vi "Set Connection Status.vi"(8 "error in (no error)":errorcluster, 10 "Connection Status":T1, 11 "S7NetCom in":refnum<class "S7NetCom.lvclass">) -> (0 "error out":errorcluster, 3 "S7NetCom out":refnum<class "S7NetCom.lvclass">)   [LabVIEW 2014, in "S7NetCom.lvclass"]
doc: "____\nCopyright (c) 2019 Hampel Software Engineering (HSE), released under BSD license. More info can be found on https://dokuwiki.hampel-soft.com/code/hse/s7netcom. Original code published by Marc Christenson, Sisu Devices."
uses:
  S7NetCom.lvclass
  Controls/S7NetCom_ConnectionStatus.ctl
  S7NetCom.lvclass/S7NetCom.ctl
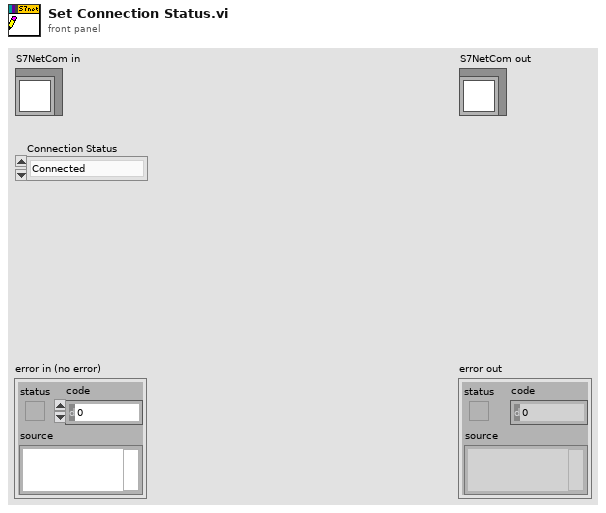
[diagram p1: front panel]
types:
  T1 = typedef "S7NetCom.lvclass/S7NetCom_ConnectionStatus.ctl" = enum16{"Connected", "Not Connected"}
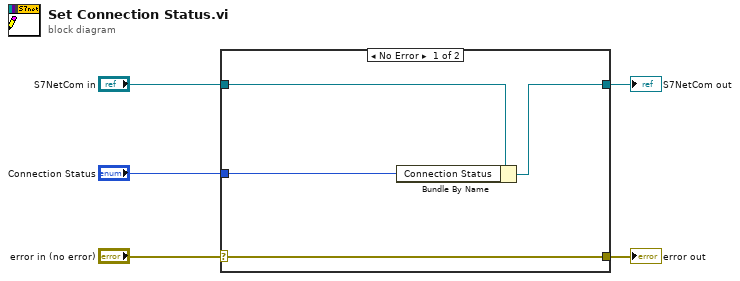
[diagram p0: block diagram]
diagram:
  n1 = case shown="No Error" "error in (no error)" {
    selector: "error in (no error)" -> [w9 w10]
    tunnel: [w9 w10] -> w4
    tunnel: [w7 w11] -> w2
    tunnel: "S7NetCom in" -> [w8 w11]
    tunnel: "Connection Status" -> [w6 _]
    frame No Error {
      n2 = Bundle By Name(cluster=w8, "Connection Status"=w6) -> (w7:refnum<class "S7NetCom.lvclass">)
    }
    frame Error {
    }
  }
  "error out" <- w4
  "S7NetCom out" <- w2
